vi "Update_VI_Controls_description.vi"(4 "ControlDetails":T1(array[cluster]), 6 "VI Description":string, 8 "error in (no error)":errorcluster, 9 "VI Ref":refnum<vi>, 10 "Control References":refnum<vi>[](array[refnum])=[refnum, refnum, refnum, refnum, refnum, refnum, refnum], 11 "Control Labels":string[](array[string])) -> (0 "error out":errorcluster)   [LabVIEW 2020, in "lv_documentation.lvlib"]
doc: "This module updates the control's labels and documentation associated with a specific control of the selected VI."
uses:
  lv_documentation.lvlib
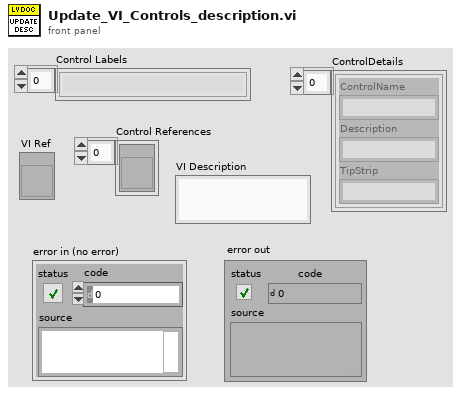
[diagram p1: front panel]
types:
  T1 = cluster{"ControlName":string, "Description":string, "TipStrip":string}[]
  T2 = cluster{"ControlName":string, "Description":string, "TipStrip":string}
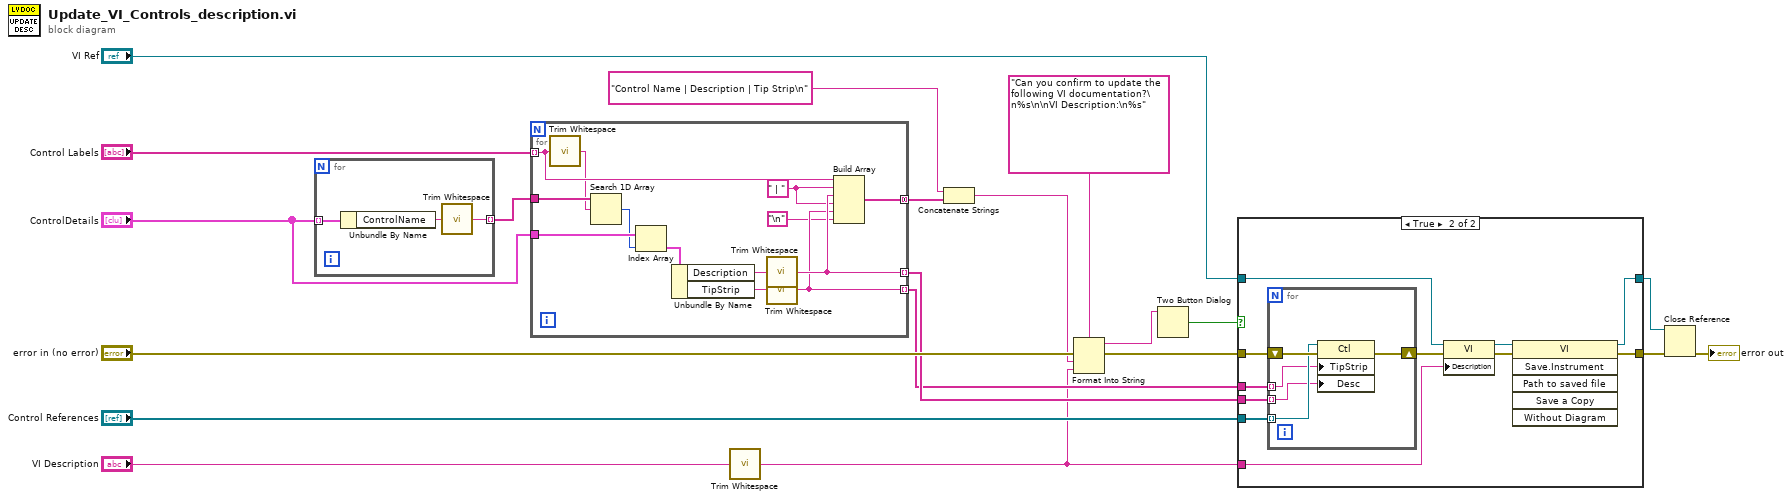
[diagram p0: block diagram]
diagram:
  n1 = for {
    tunnel: "ControlDetails" -> [w22] mode=indexing
    tunnel: [w23] -> w18 mode=indexing
    n2 = Unbundle By Name(w22) -> ("ControlName"=w21:string)
    n3 = call <vilib>:"Trim Whitespace.vi"("string"=w21) -> ("trimmed string"=w23:string)  [unwired: 1 in]
  }
  n4 = for {
    tunnel: "ControlDetails" -> [w35]
    tunnel: "Control Labels" -> [w33] mode=indexing
    tunnel: w18 -> [w36]
    tunnel: [w32] -> w9 mode=indexing
    tunnel: [w31] -> w8 mode=indexing
    tunnel: [w29] -> w16 mode=concatenating
    w30 = " | " ("element")
    n5 = call <vilib>:"Trim Whitespace.vi"("string"=w33) -> ("trimmed string"=w28:string)  [unwired: 1 in]
    n6 = Search 1D Array(1D array=w36, element=w28) -> (index of element=w34:i32)  [unwired: 1 in]
    n7 = Index Array(array=w35, index=w34) -> (element=w26:T2)
    n8 = Unbundle By Name(w26) -> ("Description"=w25:string, "TipStrip"=w24:string)
    n9 = call <vilib>:"Trim Whitespace.vi"("string"=w25) -> ("trimmed string"=w32:string)  [unwired: 1 in]
    n10 = call <vilib>:"Trim Whitespace.vi"("string"=w24) -> ("trimmed string"=w31:string)  [unwired: 1 in]
    n11 = Build Array(w33, w30, w32, w30, w31, "\n" ("delimiter")) -> (w29:string[])
  }
  n12 = call <vilib>:"Trim Whitespace.vi"("string"="VI Description") -> ("trimmed string"=w6:string)  [unwired: 1 in]
  n13 = Concatenate Strings("Control Name | Description | Tip Strip\n" ("Label.Text"), w16) -> (w13:string)
  n14 = Format Into String(format string="Can you confirm to update the following VI documentation?\n%s\n\nVI Description:\n%s", error in="error in (no error)", w13, w6) -> (resulting string=w12:string, error out=w11:errorcluster)  [unwired: 1 in]
  n15 = Two Button Dialog(message=w12) -> (T button?=w2:bool)  [unwired: 2 in]
  n16 = case shown="True" w2 {
    tunnel: w11 -> [w38 w49]
    tunnel: "Control References" -> [_ w48]
    tunnel: w9 -> [_ w47]
    tunnel: w8 -> [_ w46]
    tunnel: "VI Ref" -> [w37 w44]
    tunnel: w6 -> [_ w43]
    tunnel: [w38 w42] -> w4
    tunnel: [w37 w40] -> w3
    frame False {
    }
    frame True {
      n17 = for {
        shift-right: [w53] -> w39
        shift-left: w49 -> [w54]
        tunnel: w48 -> [w52] mode=indexing
        tunnel: w47 -> [w50] mode=indexing
        tunnel: w46 -> [w51] mode=indexing
        n18 = property class="Ctl"(reference=w52, error in=w54, "TipStrip"=w51, "Desc"=w50) -> (error out=w53:errorcluster)  [unwired: 1 out]
      }
      n19 = property class="VI"(reference=w44, error in=w39, "Description"=w43) -> (reference out=w41:refnum<vi>, error out=w45:errorcluster)
      n20 = invoke class="VI" method="Save.Instrument"(reference=w41, error in=w45) -> (reference out=w40:refnum<vi>, error out=w42:errorcluster)  [unwired: 4 in, 4 out]
    }
  }
  n21 = Close Reference(reference=w3, error in (no error)=w4) -> (error out=→"error out":errorcluster)
